vi "Encode Base58 UID.vi"(8 "Error In":errorcluster, 11 "UID":u64) -> (0 "Error Out":errorcluster, 3 "Base58 UID":string)   [LabVIEW 2011, in "Tinkerforge.lvlib"]
doc: "This VI encodes the U64 <B>UID</B> as Base58 string."
uses:
  Tinkerforge.lvlib
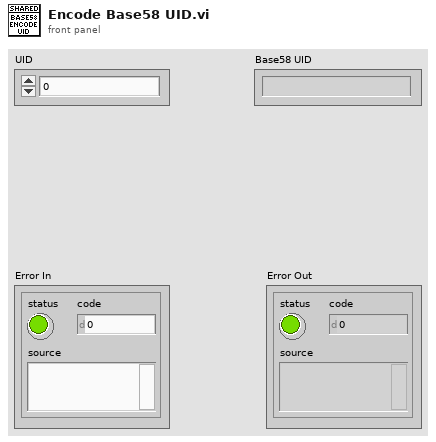
[diagram p1: front panel]
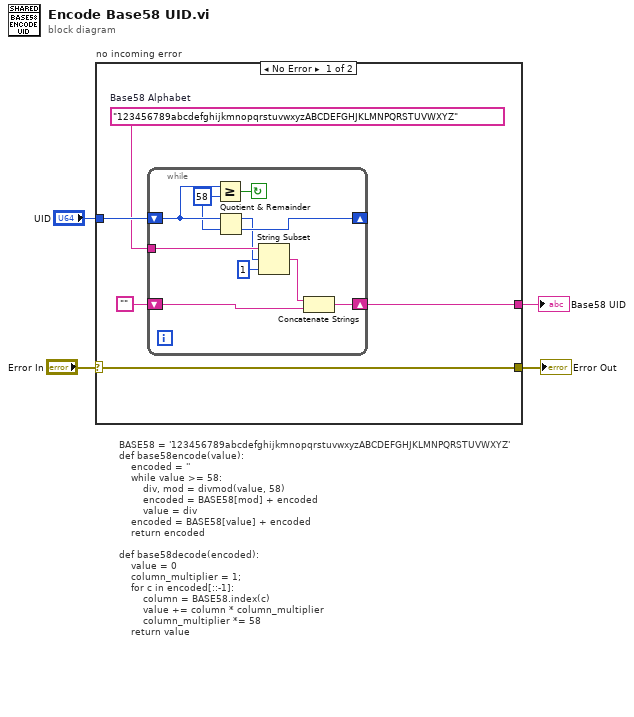
[diagram p0: block diagram]
diagram:
  # "BASE58 = '123456789abcdefghijkmnopqrstuvwxyzABCDEFGHJKLMNPQRSTUVWXYZ'\ndef base58encode(value):\n    encoded = ''\n    while value >= 58:\n        div, mod = divmod(value, 58)\n        encoded = BASE58[mod] + encoded \n        value = div\n    encoded = BASE58[value] + encoded \n    return encoded\n\ndef base58decode(encoded):\n    value = 0\n    column_multiplier = 1;\n    for c in encoded[::-1]:\n        column = BASE58.index(c)\n        value += column * column_multiplier\n        column_multiplier *= 58\n    return value"
  n1 = case "no incoming error" shown="No Error" "Error In" {
    selector: "Error In" -> [w9 w20]
    tunnel: [w9 w20] -> w3
    tunnel: "UID" -> [w8 _]
    tunnel: [w5 _] -> w1
    frame No Error {
      w6 = "123456789abcdefghijkmnopqrstuvwxyzABCDEFGHJKLMNPQRSTUVWXYZ"  # Base58 Alphabet
      n2 = while {
        shift-right: [w16] -> _
        shift-left: w8 -> [w18]
        tunnel: w6 -> [w15]
        shift-right: [w10] -> w5
        shift-left: "" -> [w12]
        stop <- w19 continue-if-true
        w17 = u64 58 ("y")
        n3 = Greater Or Equal?(x=w18, y=w17) -> (x >= y?=w19:bool)
        n4 = Quotient & Remainder(x=w18, y=w17) -> (x-y*floor(x/y)=w14:u64, floor(x/y)=w16:u64)
        n5 = String Subset(string=w15, offset (0)=w14, length (rest)=1 ("length (rest)")) -> (substring=w11:string)
        n6 = Concatenate Strings(w11, w12) -> (w10:string)
      }
    }
    frame Error {
    }
  }
  "Error Out" <- w3
  "Base58 UID" <- w1
